vi "AutoDispenseRemainder(SubVI).vi"(10 "Array of UInt16":u16[](array[numeric]), 11 "Refnum in":refnum<k20>) -> ()   [LabVIEW 2013]
uses:
  <vilib>/rvi/interface/common/niFpgaWaitOnOcc.vi
  <vilib>/Utility/error.llb/Error Cluster From Error Code.vi
  <vilib>/rvi/errors/niLvFpgaAdjustHostInterfaceError.vi
  <vilib>/rvi/interface/nirviReadWriteControl/nirviReadWriteControl.xnode
  NiFpgaLv.dll
  <vilib>/rvi/interface/Simulation/niFpgaSimulationCallBeginRW.vi
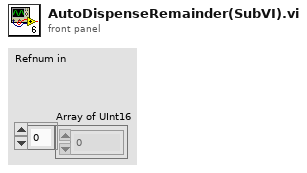
[diagram p1: front panel]
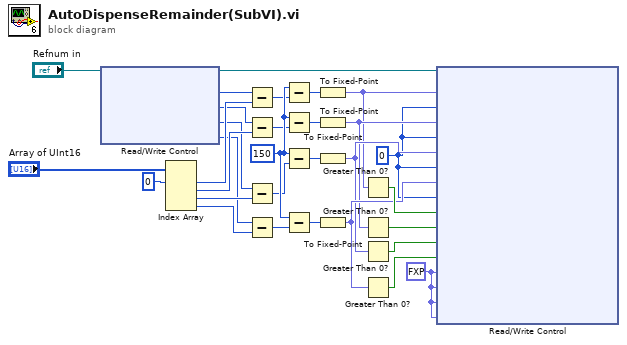
[diagram p0: block diagram]
diagram:
  w31 = u16 150 ("x")
  w12 = fxp<+,22,9> 10.0 ("Mean 4")
  w11 = i16 0 ("Automated Pellets Dispensed 2")
  n1 = xnode "Read/Write Control"("FPGA VI Reference In"="Refnum in") -> ("FPGA VI Reference Out"=w21:refnum<k20>, "Pellets Dispensed 1"=w1:i16, "Pellets Dispensed 2"=w2:i16, "Pellets Dispensed 3"=w3:i16, "Pellets Dispensed 4"=w4:i16)  [unwired: 1 in, 1 out]
  n2 = Index Array(array="Array of UInt16", index #1=0 ("index")) -> (element #1=w7:u16, element #2=w8:u16, element #3=w9:u16, element #4=w10:u16)  [unwired: 3 in]
  n3 = Subtract(x=w1, y=w7) -> (x-y=w29:u16)
  n4 = Subtract(x=w2, y=w8) -> (x-y=w27:u16)
  n5 = Subtract(x=w3, y=w9) -> (x-y=w26:u16)
  n6 = Subtract(x=w4, y=w10) -> (x-y=w23:u16)
  n7 = Subtract(x=w31, y=w29) -> (x-y=w30:u16)
  n8 = Subtract(x=w31, y=w27) -> (x-y=w28:u16)
  n9 = Subtract(x=w31, y=w26) -> (x-y=w25:u16)
  n10 = Subtract(x=w31, y=w23) -> (x-y=w24:u16)
  n11 = To Fixed-Point(number=w30) -> (fixed-point=w13:fxp<+,10,10>)  [unwired: 1 in]
  n12 = To Fixed-Point(number=w28) -> (fixed-point=w14:fxp<+,10,10>)  [unwired: 1 in]
  n13 = To Fixed-Point(number=w25) -> (fixed-point=w15:fxp<+,10,10>)  [unwired: 1 in]
  n14 = To Fixed-Point(number=w24) -> (fixed-point=w16:fxp<+,10,10>)  [unwired: 1 in]
  n15 = Greater Than 0?(x=w13) -> (x > 0?=w17:bool)
  n16 = Greater Than 0?(x=w14) -> (x > 0?=w18:bool)
  n17 = Greater Than 0?(x=w15) -> (x > 0?=w19:bool)
  n18 = Greater Than 0?(x=w16) -> (x > 0?=w20:bool)
  n19 = xnode "Read/Write Control"("FPGA VI Reference In"=w21, "Automated Pellets Target 1"=w13, "Automated Pellets Dispensed 1"=w11, "Automated Pellets Target 2"=w14, "Automated Pellets Dispensed 2"=w11, "Automated Pellets Target 3"=w15, "Automated Pellets Dispensed 3"=w11, "Automated Pellets Target 4"=w16, "Automated Pellets Dispensed 4"=w11, "Automatic Dispense 1"=w17, "Automatic Dispense 2"=w18, "Automatic Dispense 3"=w19, "Automatic Dispense 4"=w20, "Mean 1"=w12, "Mean 2"=w12, "Mean 3"=w12, "Mean 4"=w12) -> ()  [unwired: 1 in, 2 out]
